vi "纳清电导率电极校准.vi"() -> ()   [LabVIEW 2016, in "斯坦道多参数.lvlib"]
uses:
  <vilib>/Utility/miscctls.llb/LVPointTypeDef.ctl
  <vilib>/Analysis/NI_AALBase.lvlib
panel:
  out "第二点信号值":dbl
  out "第一点信号值":dbl
  out "盐度":dbl caption="盐度测量值" format="%#.2f"
  out "当前量程":u16
  out "报警信息":string
  out "通讯状态":string
  out "第二点校准值":dbl
  out "第一点校准值":dbl
  in  "校准停止":bool
  in  "校准启动":bool
  in  "校准模式":u16(ring) items=["单点校准"]
  out "最小值":sgl format="%#.2f"
  out "最大值":sgl format="%#.2f"
  out "波形图表":dbl(graph) caption="历史曲线"
  out "mean":dbl caption="均值" format="%#.2f"
  out "standard deviation":dbl caption="标准差" format="%#.2f"
  out "变异系数":dbl format="%#.6f"
  out "测量值":sgl format="%#.2f"
  out "提示":string
  out "标液1":sgl
  out "原始光强数值":sgl caption="信号值" format="%#.6f"
  out "温度":dbl format="%#.2f"
  # "电导率电极设定"
  # "℃"
  # "μS/cm"
  # "ppt"
  # "电阻"
  # "请选择校准模式:"
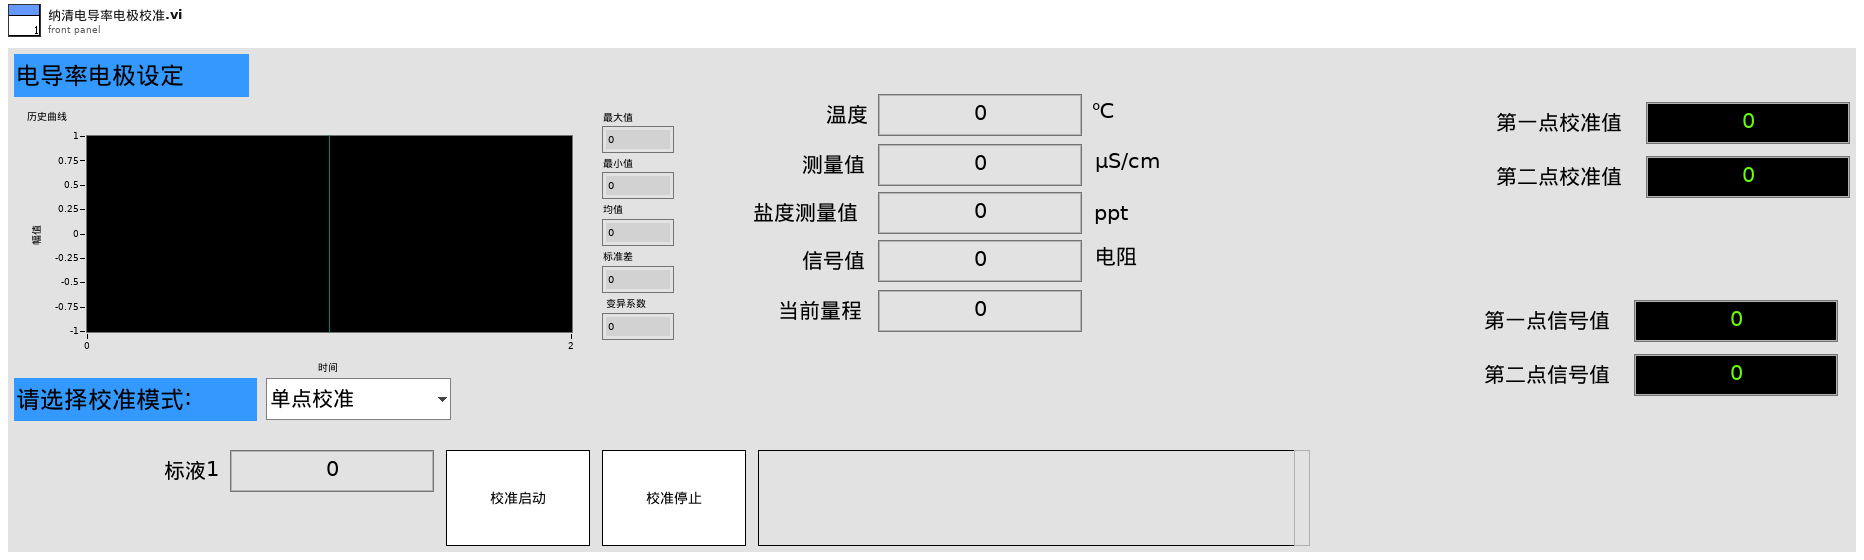
[diagram p1: front panel]
types:
  T1 = typedef "LVPointTypeDef.ctl" = cluster{"Horizontal":i16, "Vertical":i16}
  T2 = cluster{"报警码":u16, "电导率数据（uS/cm）":sgl, "0x0003 NC":sgl, "温度数据":sgl, "电导率原始信号电阻":sgl, "当前量程":u16, "温度补偿系数":sgl, "0X0009_NC":string, "产品名称":string, "序列号":string, "硬件版本":string, "软件版本":string, "通讯地址":u16, "波特率":u16, "设备类型":u16, "0X0026_NC":string, "第一点原始数据":sgl, "第一点校准数据":sgl, "0X0035_NC":sgl, "0X0037_NC":sgl, "探头校准命令":u16, "温度校准参数":sgl, "温度校准命令":u16}
  T3 = cluster{"温度测量值":sgl, "测量值":sgl, "温度偏移修正值":sgl, "信号值":sgl}
  T4 = enum8{"Enabled", "Disabled", "Disabled and Grayed Out"}
  T5 = cluster{"ph":bool, "DO":bool, "Cond":bool, "Turb":bool, "叶绿素a":bool, "藻密度":bool, "ORP":bool}
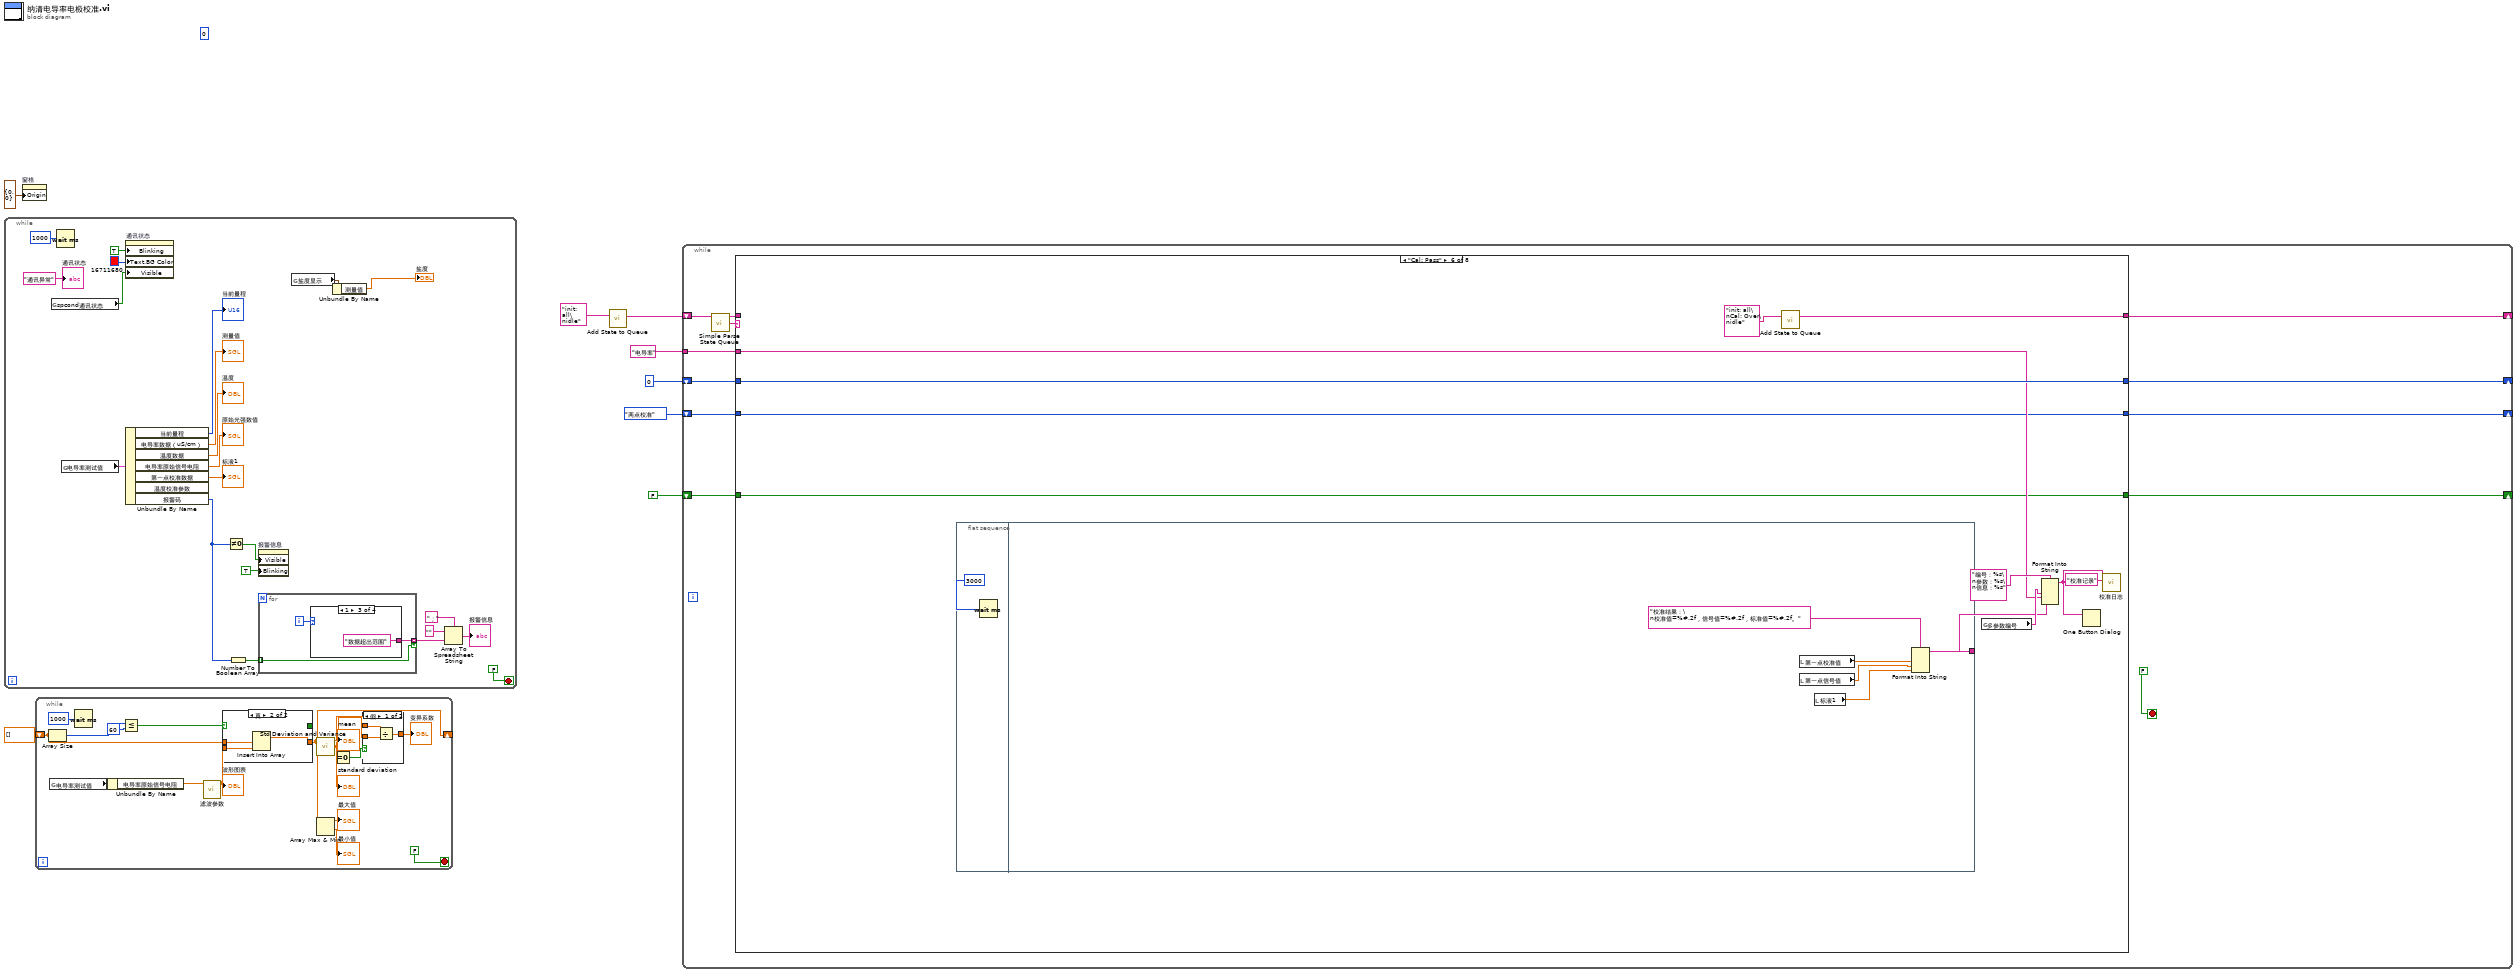
[diagram p0: block diagram]
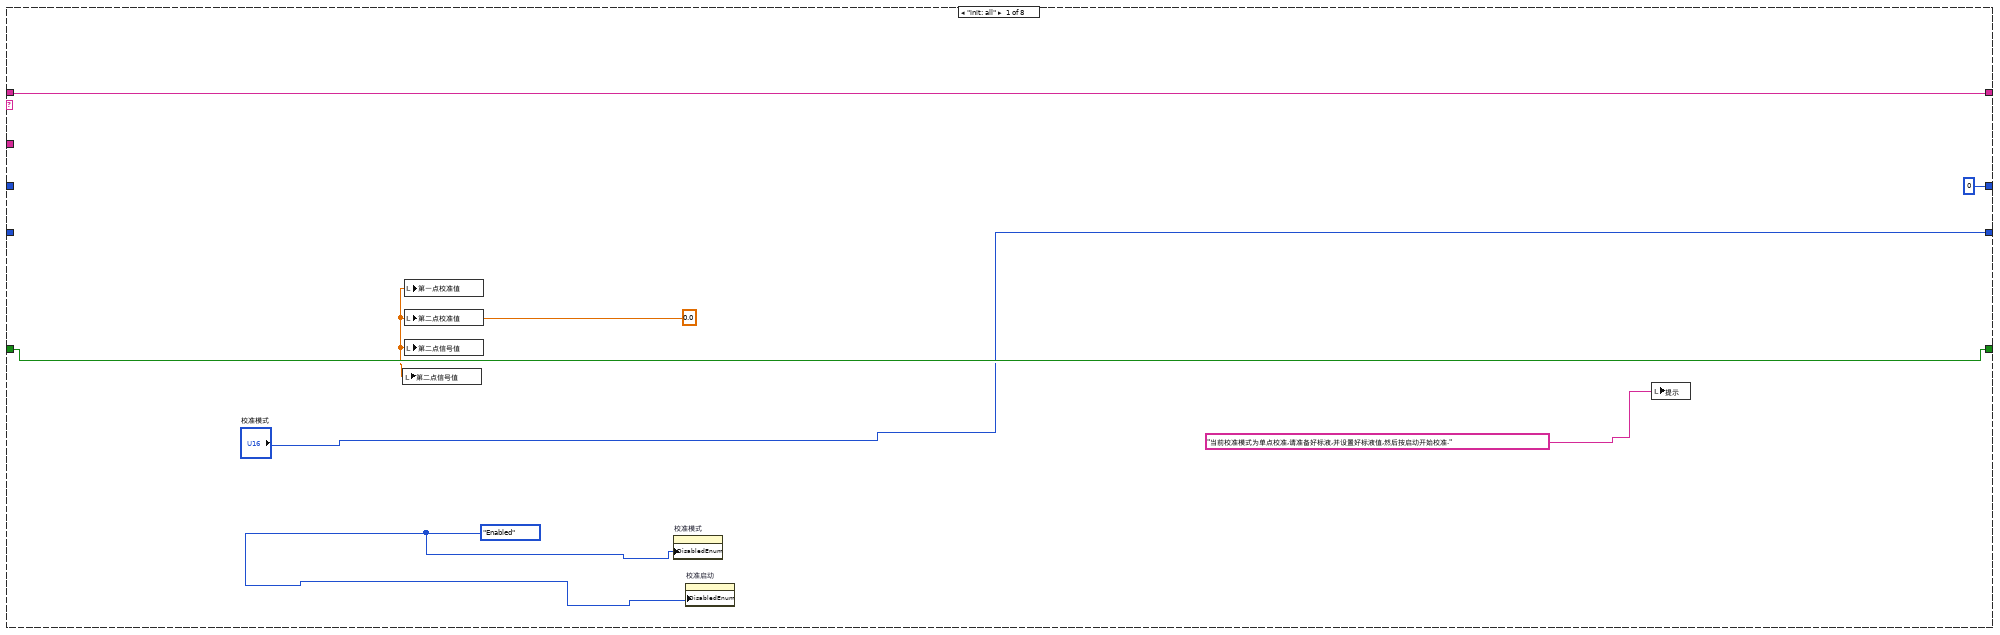
[diagram p2: hidden frame]
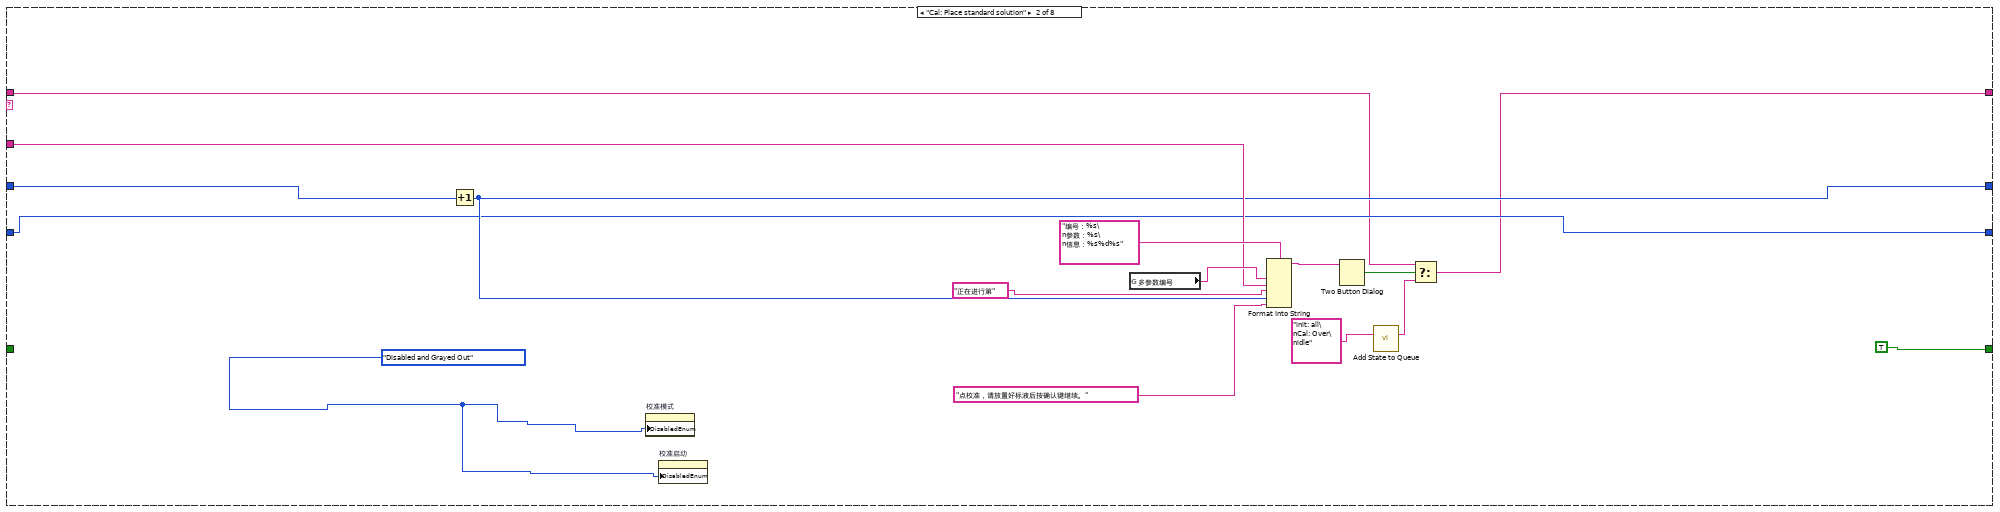
[diagram p3: hidden frame]
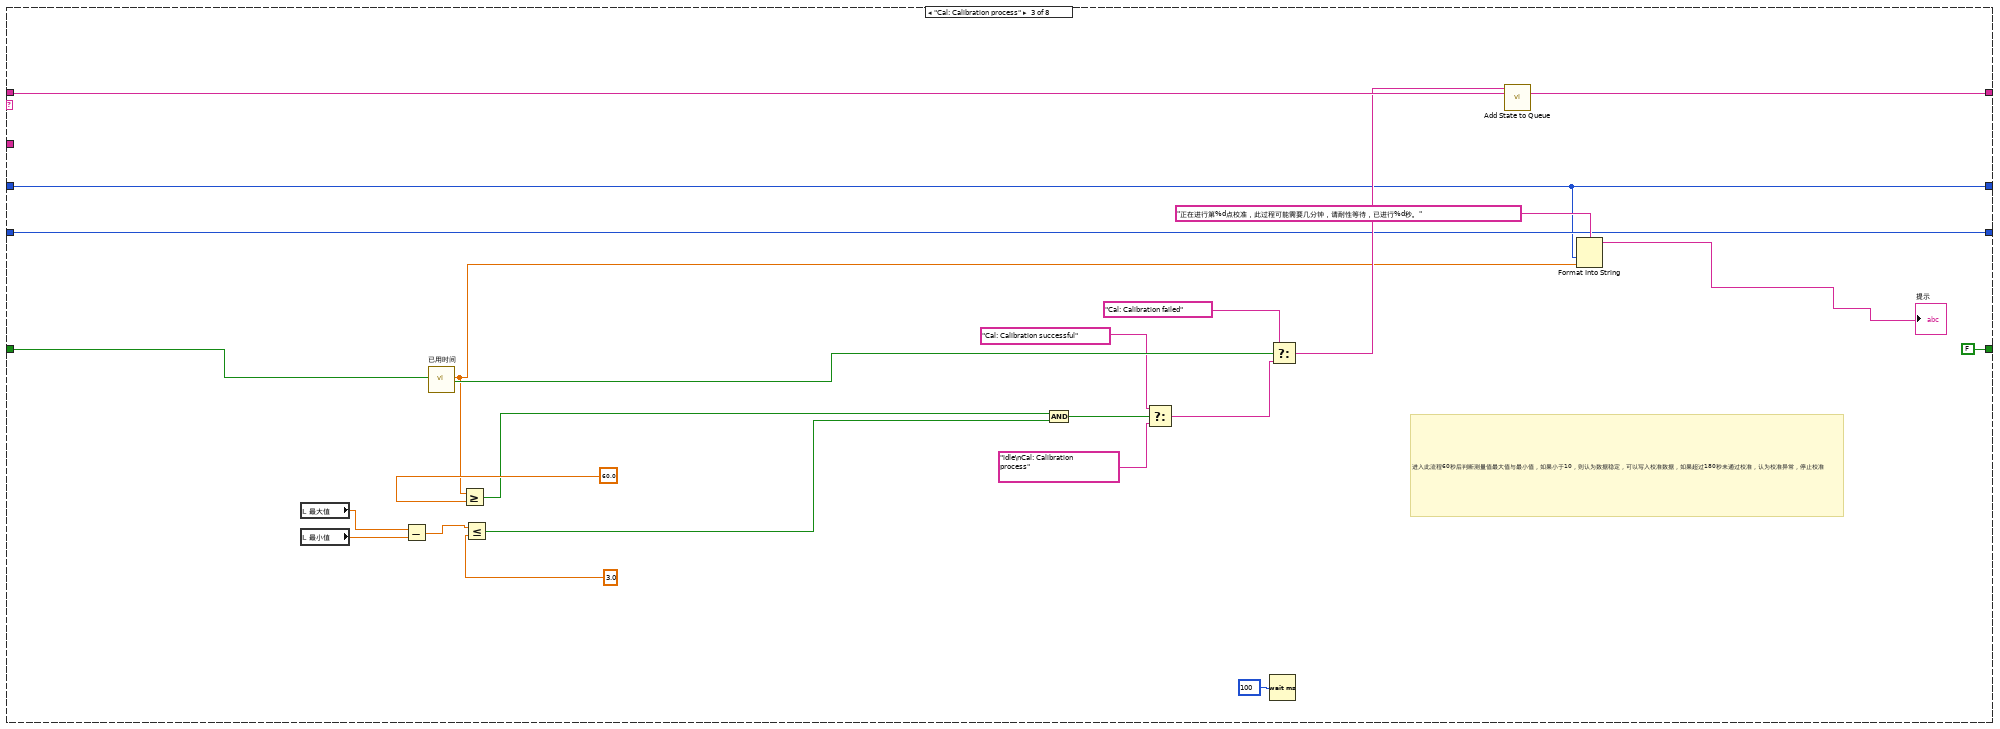
[diagram p4: hidden frame]
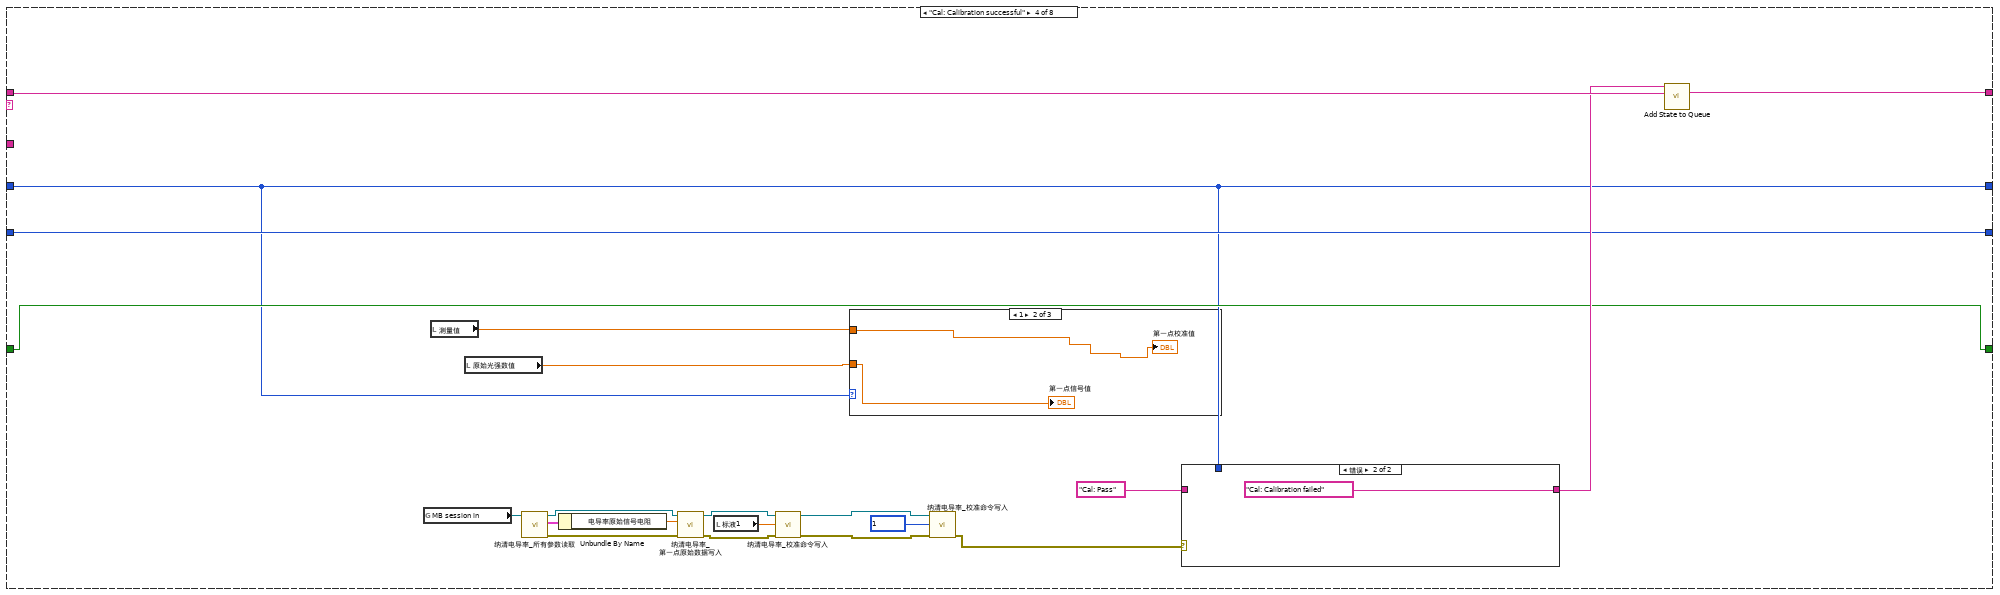
[diagram p5: hidden frame]
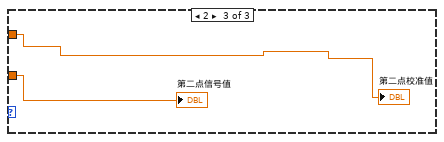
[diagram p7: hidden frame]
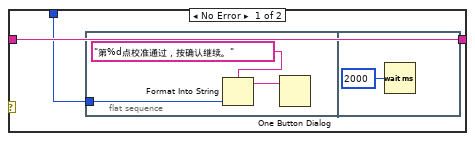
[diagram p8: hidden frame]
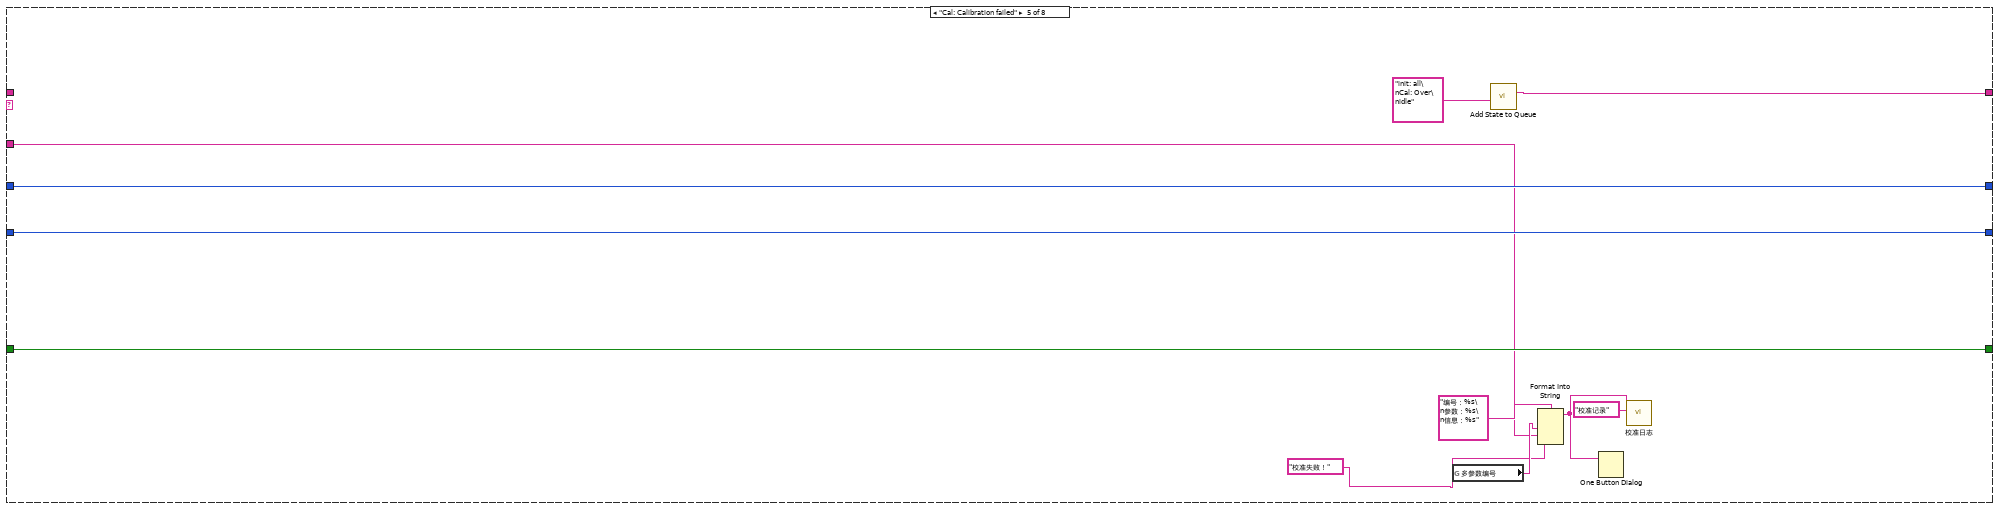
[diagram p9: hidden frame]
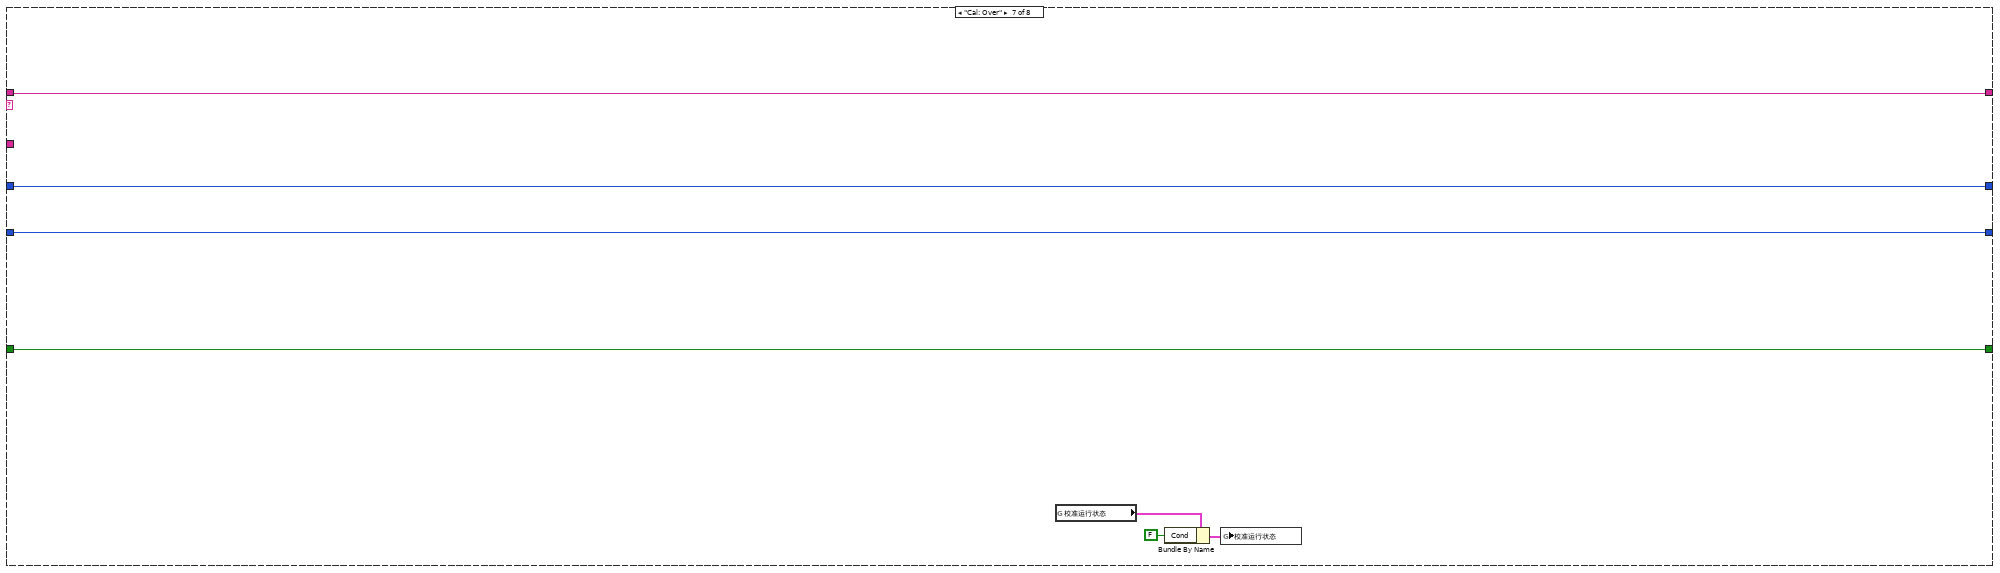
[diagram p10: hidden frame]
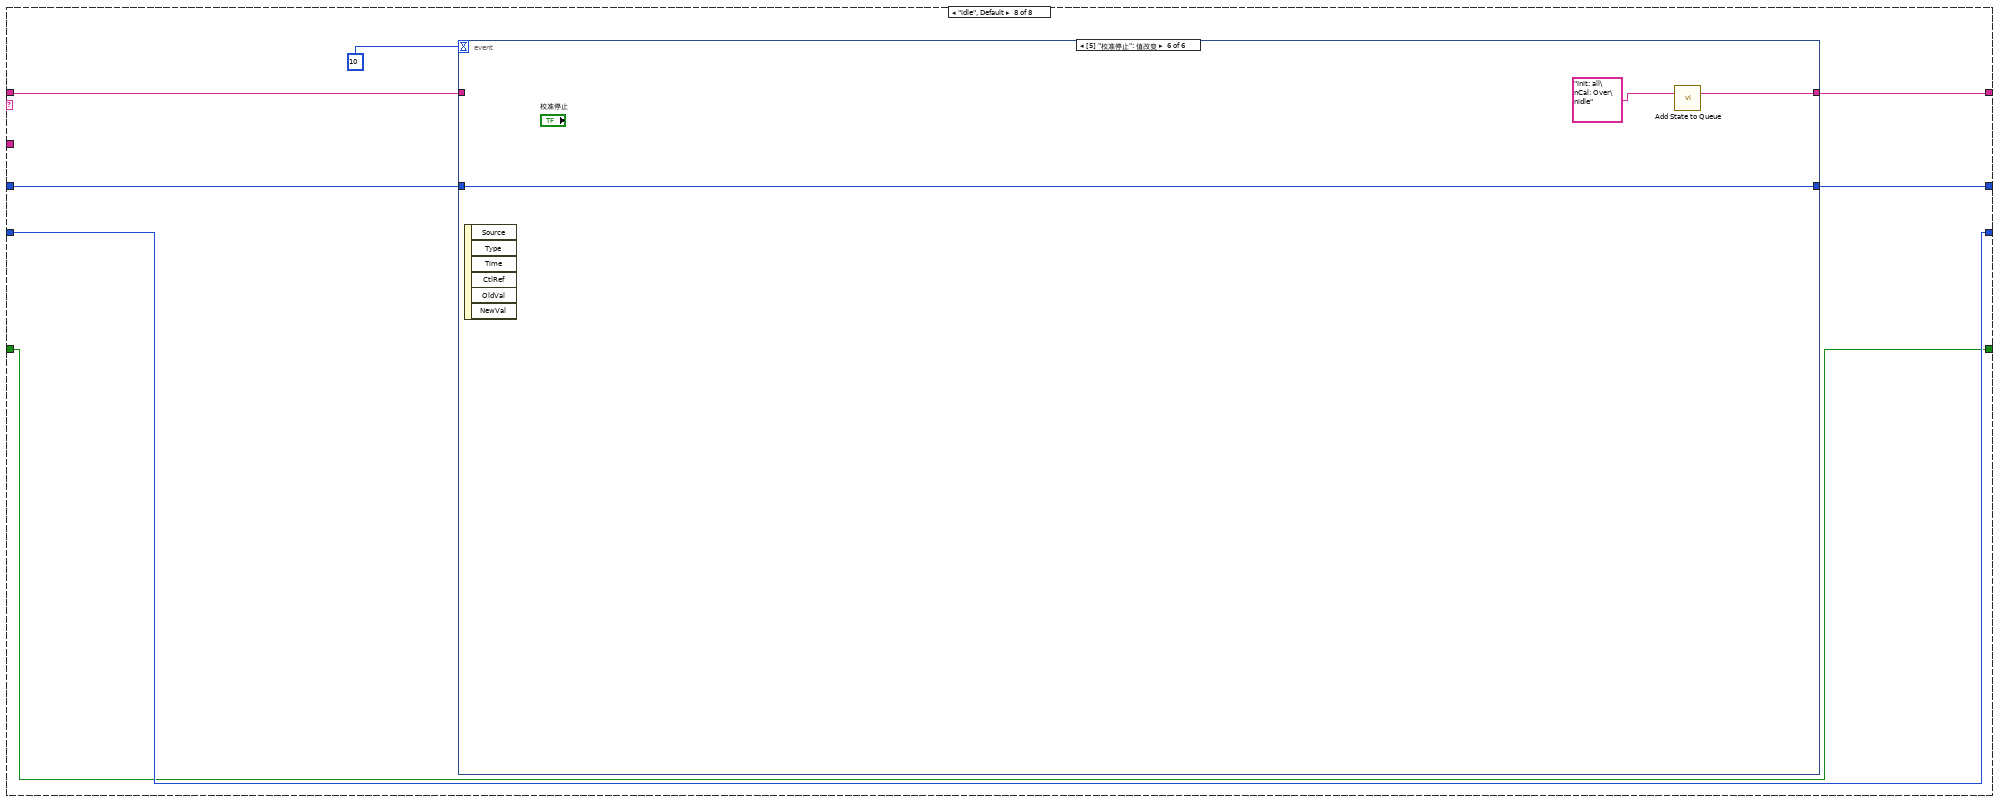
[diagram p11: hidden frame]
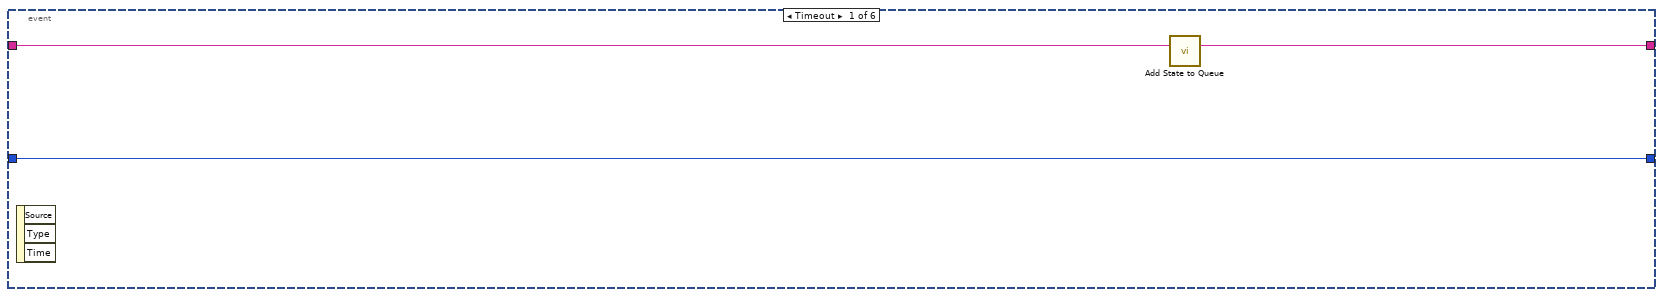
[diagram p12: hidden frame]
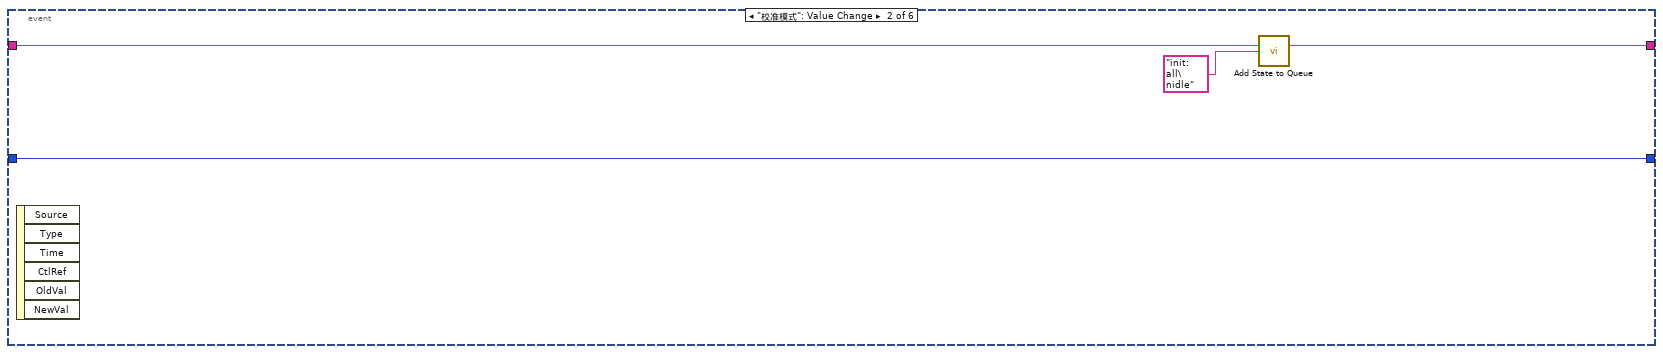
[diagram p13: hidden frame]
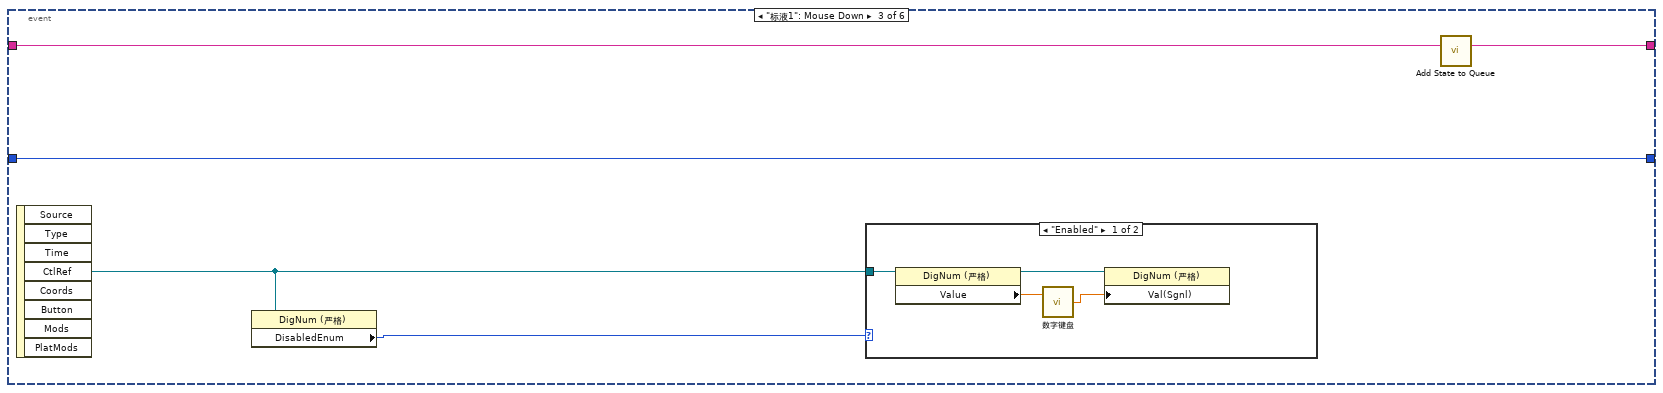
[diagram p14: hidden frame]
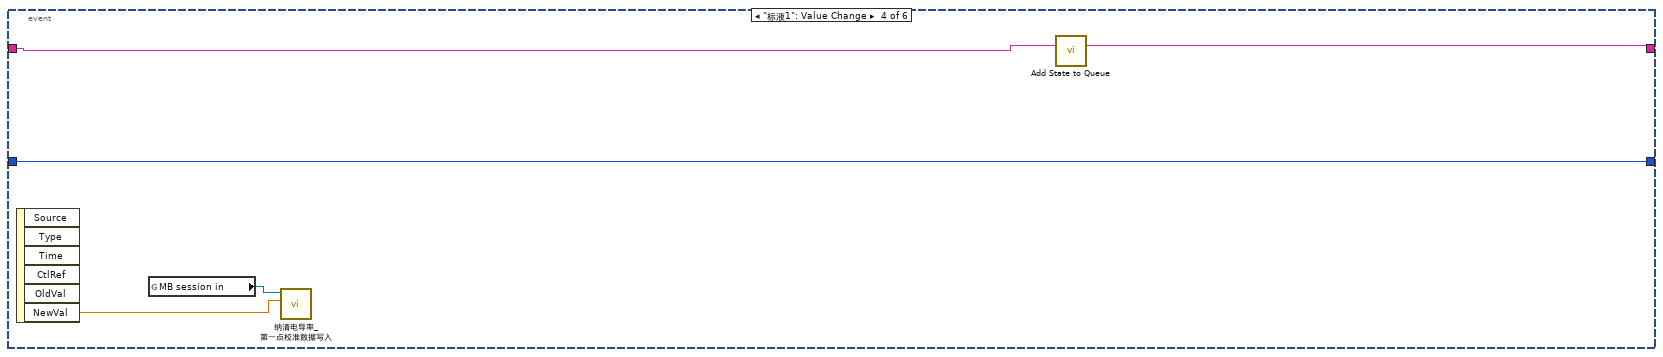
[diagram p16: hidden frame]
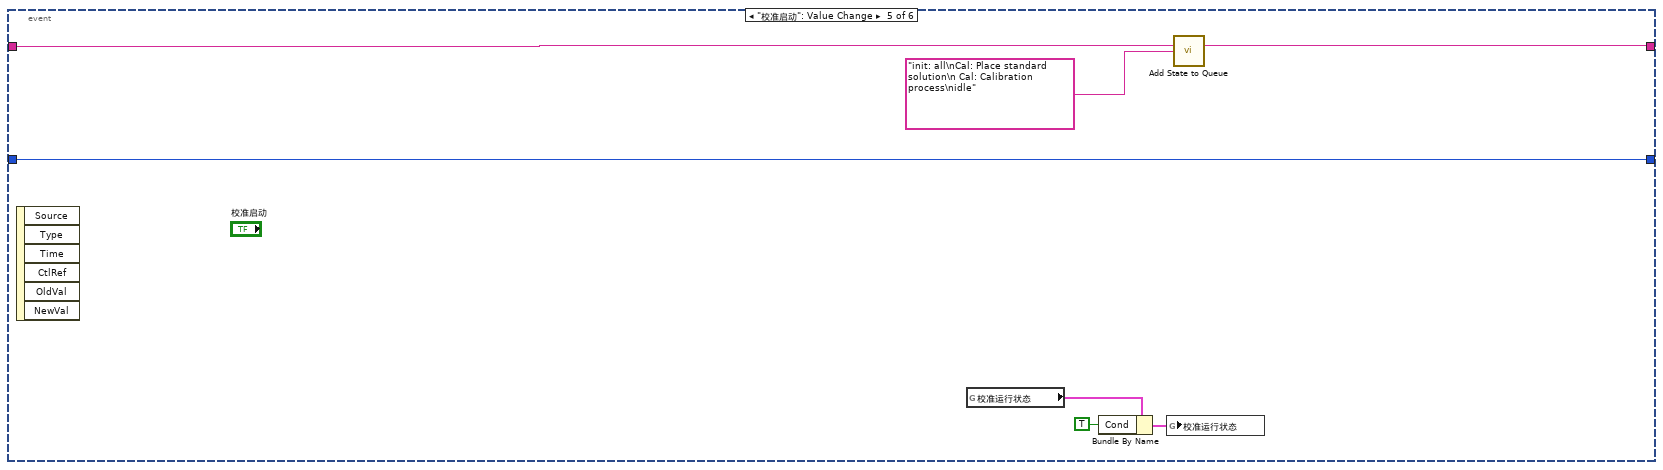
[diagram p17: hidden frame]
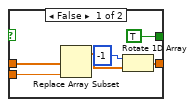
[diagram p19: hidden frame]
diagram:
  (unwired) 0
  n1 = while {
    stop <- FALSE stop-if-true
    n2 = global read "多参数全局变量.vi" "spcond通讯状态"() -> (w20:bool)
    n3 = Wait (ms)(milliseconds to wait=u32 1000 ("等待时间（毫秒）")) -> ()  [unwired: 1 out]
    n4 = global read "纳清过程全局变量.vi" "电导率测试值"() -> (w28:T2)
    n5 = property on="通讯状态" class="Str"("Blinking"=TRUE ("闪烁"), "Text.BG Color"=u32 16711680, "Visible"=w20) -> ()  [unwired: 2 in, 2 out]
    n6 = Unbundle By Name(w28) -> ("当前量程"=→"当前量程":u16, "电导率数据（uS/cm）"=→"测量值":sgl, "温度数据"=→"温度":sgl, "电导率原始信号电阻"=→"原始光强数值":sgl, "第一点校准数据"=→"标液1":sgl, "报警码"=w14:u16)  [unwired: 1 out]
    n7 = Not Equal To 0?(x=w14) -> (x != 0?=w13:bool)
    n8 = Number To Boolean Array(number=w14) -> (Boolean array=w19:bool[])
    n9 = property on="报警信息" class="Str"("Visible"=w13, "Blinking"=TRUE ("闪烁")) -> ()  [unwired: 2 in, 2 out]
    n10 = for {
      tunnel: w19 -> [w31] mode=indexing
      tunnel: [w32] -> w18 mode=indexing if=w31
      i -> [w33]
      n11 = case shown="1" w33 {
        tunnel: [_ "温度超出范围" "数据超出范围" "温度传感器故障"] -> w32
        frame Default {
        }
        frame 0 {
        }
        frame 1 {
        }
        frame 8 {
        }
      }
    }
    n12 = global read "多参数全局变量.vi" "盐度显示"() -> (w9:T3)
    n13 = Unbundle By Name(w9) -> ("测量值"=→"盐度":sgl)
    n14 = Array To Spreadsheet String(delimiter (Tab)="；" ("分隔符(Tab)"), array=w18, 3:"" ("格式字符串")) -> (spreadsheet string=→"报警信息":string)
    "通讯状态" <- "通讯异常" ("当前串口")
  }
  n15 = property on="窗格" class="Pane"("Origin"=T1 {"Horizontal"=0, "Vertical"=0} ("原点")) -> ()  [unwired: 2 in, 2 out]
  n16 = while {
    shift-right: [w42] -> _
    shift-left: sgl[] [] -> [w48]
    stop <- FALSE stop-if-true
    n17 = Array Size(array=w48) -> (size(s)=w50:i32)
    n18 = global read "纳清过程全局变量.vi" "电导率测试值"() -> (w39:T2)
    n19 = Wait (ms)(milliseconds to wait=u32 1000 ("等待时间（毫秒）")) -> ()  [unwired: 1 out]
    n20 = Unbundle By Name(w39) -> ("电导率原始信号电阻"=w38:sgl)
    n21 = Less Or Equal?(x=w50, y=60) -> (x <= y?=w49:bool)
    n22 = call "滤波参数.vi"("x"=w38) -> ("mode"=w37:dbl)  [unwired: 10 in]
    "波形图表" <- w37
    n23 = case shown="真" w49 {
      tunnel: w48 -> [w61 w64]
      tunnel: w37 -> [w59 w63]
      tunnel: [w57 w62] -> w42
      tunnel: [TRUE _] -> _
      frame False {
        n24 = Replace Array Subset(array=w61, new element=w59) -> (w60:sgl[])  [unwired: 1 in]
        n25 = Rotate 1D Array(1:w60, 2:-1 ("n")) -> (0:w57:sgl[])
      }
      frame True {
        n26 = Insert Into Array(array=w64, new element=w63) -> (w62:sgl[])  [unwired: 1 in]
      }
    }
    n27 = call <vilib>:"Std Deviation and Variance.vi"("X"=w42) -> ("mean"=w46:dbl, "standard deviation"=w45:dbl)  [unwired: 1 in, 1 out]
    "mean" <- w46
    "standard deviation" <- w45
    n28 = Array Max & Min(array=w42) -> (max value=→"最大值":sgl, min value=→"最小值":sgl)  [unwired: 2 out]
    n29 = Equal To 0?(x=w46) -> (x = 0?=w47:bool)
    n30 = case shown="假" w47 {
      tunnel: w45 -> [w55 _]
      tunnel: [w54 _] -> w44
      tunnel: w46 -> [w53 _]
      frame False {
        n31 = Divide(x=w55, y=w53) -> (x/y=w54:dbl)
      }
      frame True {
      }
    }
    "变异系数" <- w44
  }
  n32 = call "Add State to Queue.vi"("State(s) In (\"\")"="init: all\nidle" ("State(s) In (\"\")")) -> ("States Out"=w5:string)  [unwired: 14 in]
  n33 = while {
    shift-right: [w72] -> _
    shift-left: w5 -> [w76]
    shift-right: [w69] -> _
    shift-left: 0 -> [w71]
    tunnel: "电导率" ("State(s) In (\"\")") -> [w70]
    shift-right: [w67] -> _
    shift-left: enum16{"两点校准", "单点校准"}."两点校准" ("校准模式") -> [w68]
    shift-right: [w65] -> _
    shift-left: FALSE -> [w66]
    stop <- FALSE stop-if-true
    n34 = call "Simple Parse State Queue.vi"("State Queue"=w76) -> ("Remain States"=w73:string, "Next State"=w74:string)  [unwired: 13 in]
    n35 = case shown="\"Cal: Pass\"" w74 {
      tunnel: w73 -> [w83 w86 w118 w143 _ _ w190 w197]
      tunnel: [w83 w85 w117 w142 w163 w167 w190 w196] -> w72
      tunnel: w71 -> [_ w95 w102 w125 w166 w177 w189 w194]
      tunnel: w70 -> [_ w96 _ _ w156 w173 _ _]
      tunnel: [0 w93 w102 w125 w166 w177 w189 w195] -> w69
      tunnel: w68 -> [_ w92 w103 w137 w165 w169 w188 w193]
      tunnel: ["校准模式" w92 w103 w137 w165 w169 w188 w193] -> w67
      tunnel: w66 -> [w80 _ w105 w138 w164 w172 w187 w191]
      tunnel: [w80 TRUE FALSE w138 w164 w172 w187 w191] -> w65
      frame "init: all" {
        w77 = T4."Enabled" ("禁用")
        w79 = 0.0 ("第一点校准值")
        n36 = local write "第二点信号值"(w79) -> ()
        n37 = local write "第一点校准值"(w79) -> ()
        n38 = local write "第二点校准值"(w79) -> ()
        n39 = local write "第二点信号值"(w79) -> ()
        n40 = property on="校准模式" class="Ring (严格)"("DisabledEnum"=w77) -> ()  [unwired: 2 in, 2 out]
        n41 = property on="校准启动" class="Bool"("DisabledEnum"=w77) -> ()  [unwired: 2 in, 2 out]
        n42 = local write "提示"("当前校准模式为单点校准,请准备好标液,并设置好标液值,然后按启动开始校准." ("提示")) -> ()
      }
      frame "Cal: Place standard solution" {
        w84 = T4."Disabled and Grayed Out" ("禁用")
        n43 = Increment(x=w95) -> (x+1=w93:i32)
        n44 = property on="校准模式" class="Ring (严格)"("DisabledEnum"=w84) -> ()  [unwired: 2 in, 2 out]
        n45 = property on="校准启动" class="Bool"("DisabledEnum"=w84) -> ()  [unwired: 2 in, 2 out]
        n46 = global read "多参数全局变量.vi" "多参数编号"() -> (w98:string)
        n47 = Format Into String(format string="编号：%s\n参数：%s\n信息：%s%d%s" ("格式字符串"), w98, w96, "正在进行第" ("消息"), w93, "点校准，请放置好标液后按确认键继续。" ("消息")) -> (resulting string=w90:string)  [unwired: 2 in, 1 out]
        n48 = Two Button Dialog(message=w90) -> (T button?=w89:bool)  [unwired: 2 in]
        n49 = call "Add State to Queue.vi"("State(s) In (\"\")"="init: all\nCal: Over\nidle" ("State(s) In (\"\")")) -> ("States Out"=w87:string)  [unwired: 14 in]
        n50 = Select(t=w86, s=w89, f=w87) -> (s? t:f=w85:string)
      }
      frame "Cal: Calibration process" {
        # "进入此流程60秒后判断测量值最大值与最小值，如果小于10，则认为数据稳定，可以写入校准数据，如果超过180秒未通过校准，认为校准异常，停止校准"
        n51 = local read "最大值"() -> (w122:sgl)
        n52 = local read "最小值"() -> (w121:sgl)
        n53 = Subtract(x=w122, y=w121) -> (x-y=w123:sgl)
        n54 = call "已用时间"("Reset"=w105) -> ("Elapsed Time (s)"=w101:dbl, "Time has Elapsed"=w119:bool)  [unwired: 11 in, 6 out]
        n55 = Greater Or Equal?(x=w101, y=60.0) -> (x >= y?=w114:bool)
        n56 = Less Or Equal?(x=w123, y=3.0) -> (x <= y?=w110:bool)
        n57 = And(x=w114, y=w110) -> (x .and. y?=w111:bool)
        n58 = Select(t="Cal: Calibration successful" ("State(s) In (\"\")"), s=w111, f="idle\nCal: Calibration process" ("State(s) In (\"\")")) -> (s? t:f=w109:string)
        n59 = Wait (ms)(milliseconds to wait=u32 100 ("等待时间（毫秒）")) -> ()  [unwired: 1 out]
        n60 = Select(t="Cal: Calibration failed" ("State(s) In (\"\")"), s=w119, f=w109) -> (s? t:f=w108:string)
        n61 = call "Add State to Queue.vi"("State(s) In Front (\"\")"=w108, "State(s) In (\"\")"=w118) -> ("States Out"=w117:string)  [unwired: 13 in]
        n62 = Format Into String(format string="正在进行第%d点校准，此过程可能需要几分钟，请耐性等待，已进行%d秒。" ("格式字符串"), w102, w101) -> (resulting string=→"提示":string)  [unwired: 2 in, 1 out]
      }
      frame "Cal: Calibration successful" {
        n63 = global read "多参数全局变量.vi" "MB session in"() -> (w129:refnum<class "MB_Master.lvclass">)
        n64 = local read "测量值"() -> (w139:sgl)
        n65 = local read "原始光强数值"() -> (w140:sgl)
        n66 = call "纳清电导率_所有参数读取.vi"("MB session in"=w129) -> ("error out"=w127:errorcluster, "输出值"=w130:T2, "MB session out"=w128:refnum<class "MB_Master.lvclass">)  [unwired: 8 in]
        n67 = Unbundle By Name(w130) -> ("电导率原始信号电阻"=w131:sgl)
        n68 = call "纳清电导率_第一点原始数据写入.vi"("error in (no error)"=w127, "数值"=w131, "MB session in"=w128) -> ("error out"=w132:errorcluster, "MB session out"=w133:refnum<class "MB_Master.lvclass">)  [unwired: 7 in]
        n69 = local read "标液1"() -> (w136:sgl)
        n70 = call "纳清电导率_校准命令写入.vi"("error in (no error)"=w132, "数值"=w136, "MB session in"=w133) -> ("error out"=w134:errorcluster, "MB session out"=w135:refnum<class "MB_Master.lvclass">)  [unwired: 7 in]
        n71 = case shown="1" w125 {
          tunnel: w140 -> [_ w146 w148]
          tunnel: w139 -> [_ w145 w147]
          frame 0, Default {
          }
          frame 1 {
            "第一点信号值" <- w146
            "第一点校准值" <- w145
          }
          frame 2 {
            "第二点信号值" <- w148
            "第二点校准值" <- w147
          }
        }
        n72 = call "纳清电导率_校准命令写入.vi"("error in (no error)"=w134, "数值"=u16 1 ("starting address"), "MB session in"=w135) -> ("error out"=w124:errorcluster)  [unwired: 7 in, 1 out]
        n73 = case shown="错误" w124 {
          tunnel: "Cal: Pass" ("State(s) In (\"\")") -> [w150 _]
          tunnel: [w150 "Cal: Calibration failed" ("State(s) In (\"\")")] -> w141
          tunnel: w125 -> [w149 _]
          frame No Error {
            n74 = flat-sequence {
              tunnel: w149 -> [w151]
              frame #0 {
                n75 = Format Into String(format string="第%d点校准通过，按确认继续。" ("格式字符串"), w151) -> (resulting string=w153:string)  [unwired: 2 in, 1 out]
                n76 = One Button Dialog(message=w153) -> ()  [unwired: 1 in, 1 out]
              }
              frame #1 {
                n77 = Wait (ms)(milliseconds to wait=u32 2000 ("等待时间（毫秒）")) -> ()  [unwired: 1 out]
              }
            }
          }
          frame Error {
          }
        }
        n78 = call "Add State to Queue.vi"("State(s) In Front (\"\")"=w141, "State(s) In (\"\")"=w143) -> ("States Out"=w142:string)  [unwired: 13 in]
      }
      frame "Cal: Calibration failed" {
        n79 = global read "多参数全局变量.vi" "多参数编号"() -> (w159:string)
        n80 = call "Add State to Queue.vi"("State(s) In (\"\")"="init: all\nCal: Over\nidle" ("State(s) In (\"\")")) -> ("States Out"=w163:string)  [unwired: 14 in]
        n81 = Format Into String(format string="编号：%s\n参数：%s\n信息：%s" ("格式字符串"), w159, w156, "校准失败！" ("消息")) -> (resulting string=w158:string)  [unwired: 2 in, 1 out]
        n82 = One Button Dialog(message=w158) -> ()  [unwired: 1 in, 1 out]
        n83 = call "校准日志.vi"("table"="校准记录", "日志信息"=w158) -> ()  [unwired: 9 in, 1 out]
      }
      frame "Cal: Pass" {
        n84 = flat-sequence {
          tunnel: [w183] -> w170
          frame #0 {
            n85 = Wait (ms)(milliseconds to wait=u32 3000 ("等待时间（毫秒）")) -> ()  [unwired: 1 out]
          }
          frame #1 {
            n86 = local read "第一点校准值"() -> (w182:dbl)
            n87 = local read "第一点信号值"() -> (w180:dbl)
            n88 = local read "标液1"() -> (w179:sgl)
            n89 = Format Into String(format string="校准结果：\n校准值=%#.2f，信号值=%#.2f，标准值=%#.2f。" ("提示"), w182, w180, w179) -> (resulting string=w183:string)  [unwired: 2 in, 1 out]
          }
        }
        n90 = call "Add State to Queue.vi"("State(s) In (\"\")"="init: all\nCal: Over\nidle" ("State(s) In (\"\")")) -> ("States Out"=w167:string)  [unwired: 14 in]
        n91 = global read "多参数全局变量.vi" "多参数编号"() -> (w174:string)
        n92 = Format Into String(format string="编号：%s\n参数：%s\n信息：%s" ("格式字符串"), w174, w173, w170) -> (resulting string=w171:string)  [unwired: 2 in, 1 out]
        n93 = One Button Dialog(message=w171) -> ()  [unwired: 1 in, 1 out]
        n94 = call "校准日志.vi"("table"="校准记录", "日志信息"=w171) -> ()  [unwired: 9 in, 1 out]
      }
      frame "Cal: Over" {
        n95 = global read "多参数全局变量.vi" "校准运行状态"() -> (w185:T5)
        n96 = Bundle By Name(cluster=w185, "Cond"=FALSE) -> (w186:T5)
        n97 = global write "多参数全局变量.vi" "校准运行状态"(w186) -> ()
      }
      frame "idle", Default {
        n98 = event shown="[5] \"校准停止\": 值改变" {
          selector: _ -> [_ _ _ _ _ _]
          dyn-events: _ -> [_ _ _ _ _ _]
          timeout: 10 -> [_ _ _ _ _ _]
          tunnel: w197 -> [w200 w204 w207 w214 w225 _]
          tunnel: [w199 w203 w208 w218 w224 w227] -> w196
          tunnel: [w198 w201 w209 w217 w222 w228] -> w195
          tunnel: w194 -> [w198 w201 w209 w217 w222 w228]
          event Timeout {
            n99 = event-data() -> ()  [unwired: 1 in, 3 out]
            n100 = call "Add State to Queue.vi"("State(s) In (\"\")"=w200) -> ("States Out"=w199:string)  [unwired: 14 in]
          }
          event "校准模式": Value Change {
            n101 = event-data() -> ()  [unwired: 1 in, 6 out]
            n102 = call "Add State to Queue.vi"("State(s) In (\"\")"=w204, "State(s) At Back (\"\")"="init: all\nidle" ("State(s) In (\"\")")) -> ("States Out"=w203:string)  [unwired: 13 in]
          }
          event "标液1": Mouse Down {
            n103 = event-data() -> ("CtlRef"=w206:refnum<vi>)  [unwired: 1 in, 7 out]
            n104 = property class="DigNum (严格)"(reference=w206) -> ("DisabledEnum"=w205:T4)  [unwired: 1 in, 2 out]
            n105 = case shown="\"Enabled\"" w205 {
              tunnel: w206 -> [w213 _]
              frame "Enabled" {
                n106 = property class="DigNum (严格)"(reference=w213) -> (reference out=w210:refnum<vi>, "Value"=w211:sgl)  [unwired: 1 in, 1 out]
                n107 = call "数字键盘.vi"("OldNumber"=w211) -> ("NewNumber"=w212:dbl)  [unwired: 1 in]
                n108 = property class="DigNum (严格)"(reference=w210, "Val(Sgnl)"=w212) -> ()  [unwired: 1 in, 2 out]
              }
              frame "Disabled", Default {
              }
            }
            n109 = call "Add State to Queue.vi"("State(s) In (\"\")"=w207) -> ("States Out"=w208:string)  [unwired: 14 in]
          }
          event "标液1": Value Change {
            n110 = event-data() -> ("NewVal"=w215:sgl)  [unwired: 1 in, 5 out]
            n111 = global read "多参数全局变量.vi" "MB session in"() -> (w216:refnum<class "MB_Master.lvclass">)
            n112 = call "纳清电导率_第一点校准数据写入.vi"("数值"=w215, "MB session in"=w216) -> ()  [unwired: 8 in, 2 out]
            n113 = call "Add State to Queue.vi"("State(s) In (\"\")"=w214) -> ("States Out"=w218:string)  [unwired: 14 in]
          }
          event "校准启动": Value Change {
            n114 = event-data() -> ()  [unwired: 1 in, 6 out]
            n115 = global read "多参数全局变量.vi" "校准运行状态"() -> (w220:T5)
            n116 = Bundle By Name(cluster=w220, "Cond"=TRUE) -> (w221:T5)
            n117 = global write "多参数全局变量.vi" "校准运行状态"(w221) -> ()
            n118 = call "Add State to Queue.vi"("State(s) In (\"\")"=w225, "State(s) At Back (\"\")"="init: all\nCal: Place standard solution\n Cal: Calibration process\nidle" ("State(s) In (\"\")")) -> ("States Out"=w224:string)  [unwired: 13 in]
          }
          event "校准停止": Value Change {
            n119 = event-data() -> ()  [unwired: 1 in, 6 out]
            n120 = call "Add State to Queue.vi"("State(s) In (\"\")"="init: all\nCal: Over\nidle" ("State(s) In (\"\")")) -> ("States Out"=w227:string)  [unwired: 14 in]
          }
        }
      }
    }
  }
